vi "读取-客户单位对象集.vi"(8 "error in (no error)":errorcluster caption="错误输入（无错误）", 11 "个人剂量仪-云服务器输入":refnum<class "个人剂量仪-云服务器.lvclass">) -> (0 "error out":errorcluster caption="错误输出", 2 "客户单位对象集":refnum<class "客户单位.lvclass">[](array[class]), 3 "个人剂量仪-云服务器输出":refnum<class "个人剂量仪-云服务器.lvclass">)   [LabVIEW 2013, in "个人剂量仪-云服务器.lvclass"]
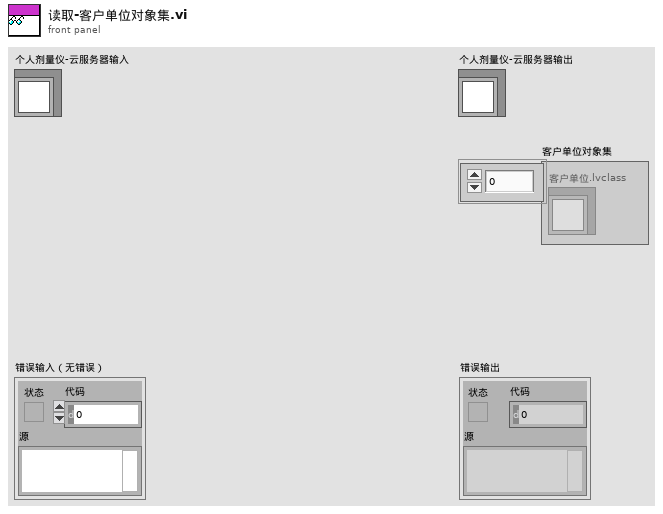
[diagram p1: front panel]
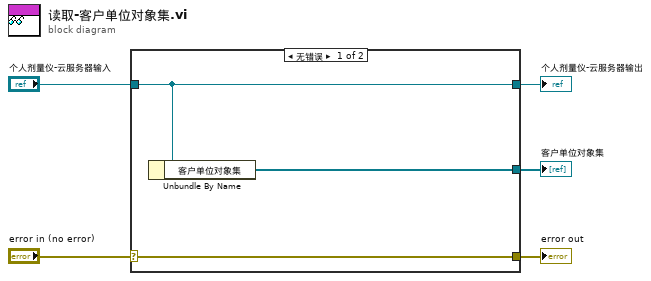
[diagram p0: block diagram]
diagram:
  n1 = case shown="无错误" "error in (no error)" {
    selector: "error in (no error)" -> [w8 w9]
    tunnel: [w8 w9] -> w4
    tunnel: [w7 w10] -> w2
    tunnel: "个人剂量仪-云服务器输入" -> [w7 w10]
    tunnel: [w6 _] -> w1
    frame No Error {
      n2 = Unbundle By Name(w7) -> ("客户单位对象集"=w6:refnum<class "客户单位.lvclass">[])
    }
    frame Error {
    }
  }
  "error out" <- w4
  "个人剂量仪-云服务器输出" <- w2
  "客户单位对象集" <- w1
